vi "流程固件设置对话框.vi"() -> ()   [LabVIEW 2022 SP3, in "斯坦道CODcr.lvlib"]
uses:
  <vilib>/Utility/miscctls.llb/LVPointTypeDef.ctl
panel:
  in  "关键参数查询":bool
  in  "仪器公式":bool
  in  "备用系数":bool
  in  "关闭心跳包":bool
  in  "参数设置":bool
  in  "修改系列号":bool
  in  "关闭":bool
  in  "外设设置":bool
  in  "固件升级":bool
  in  "流程写入":bool
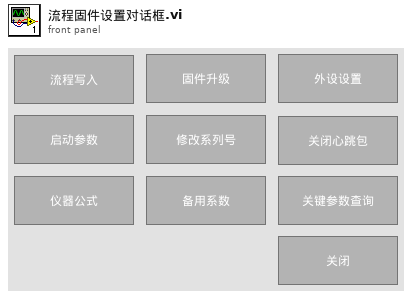
[diagram p1: front panel]
types:
  T1 = enum32{"Invalid", "Standard", "Closed", "Hidden", "Minimized", "Maximized"}
  T2 = typedef "LVPointTypeDef.ctl" = cluster{"Horizontal":i16, "Vertical":i16}
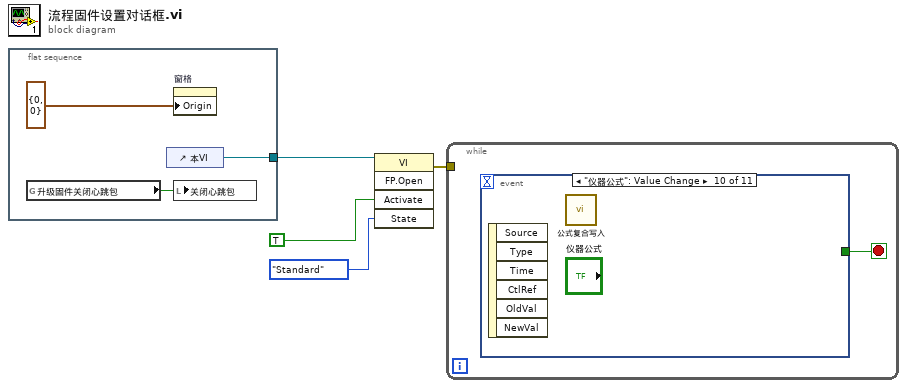
[diagram p0: block diagram]
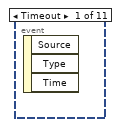
[diagram p2: hidden frame]
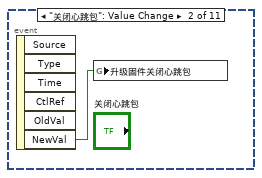
[diagram p3: hidden frame]
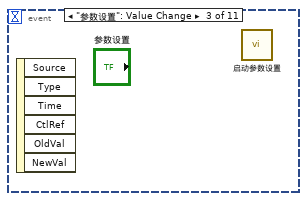
[diagram p4: hidden frame]
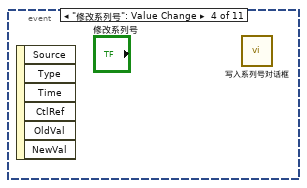
[diagram p5: hidden frame]
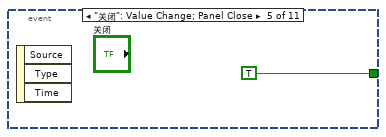
[diagram p6: hidden frame]
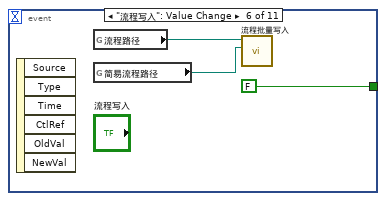
[diagram p7: hidden frame]
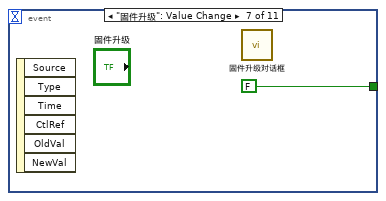
[diagram p8: hidden frame]
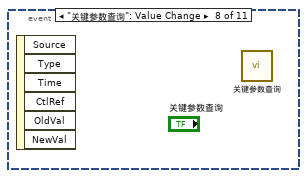
[diagram p9: hidden frame]
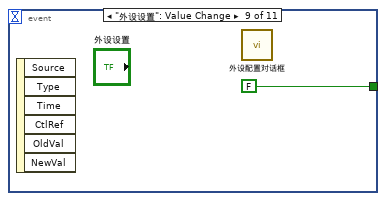
[diagram p10: hidden frame]
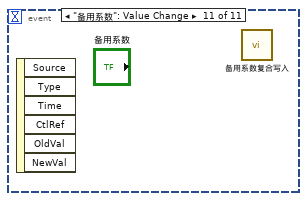
[diagram p11: hidden frame]
diagram:
  n1 = flat-sequence {
    tunnel: [w5] -> w4
    frame #0 {
      n2 = global read "VAR总磷总氮全局变量.vi" "升级固件关闭心跳包"() -> (w6:bool)
      n3 = control-ref of="本VI"() -> (w5:refnum<vi>)
      n4 = property on="窗格" class="Pane"("Origin"=T2 {"Horizontal"=0, "Vertical"=0} ("原点")) -> ()  [unwired: 2 in, 2 out]
      n5 = local write "关闭心跳包"(w6) -> ()
    }
  }
  n6 = invoke class="VI" method="FP.Open"(reference=w4, "Activate"=TRUE ("激活？"), "State"=T1."Standard" ("状态")) -> (error out=w1:errorcluster)  [unwired: 2 in, 4 out]
  n7 = while {
    tunnel: w1 -> [_]
    stop <- w8 stop-if-true
    n8 = event shown="[9] \"仪器公式\": Value Change" {
      selector: _ -> [_ _ _ _ _ _ _ _ _ _ _]
      dyn-events: _ -> [_ _ _ _ _ _ _ _ _ _ _]
      timeout: _ -> [_ _ _ _ _ _ _ _ _ _ _]
      tunnel: [_ _ _ _ TRUE FALSE FALSE _ FALSE _ _] -> w8
      event Timeout {
        n9 = event-data() -> ()  [unwired: 1 in, 3 out]
      }
      event "关闭心跳包": Value Change {
        n10 = event-data() -> ("NewVal"=w9:bool)  [unwired: 1 in, 5 out]
        n11 = global write "VAR总磷总氮全局变量.vi" "升级固件关闭心跳包"(w9) -> ()
      }
      event "参数设置": Value Change {
        n12 = event-data() -> ()  [unwired: 1 in, 6 out]
        n13 = call "启动参数设置.vi"() -> ()  [unwired: 12 in]
      }
      event "修改系列号": Value Change {
        n14 = event-data() -> ()  [unwired: 1 in, 6 out]
        n15 = call "写入系列号对话框.vi"() -> ()  [unwired: 12 in]
      }
      event "关闭": Value Change; Panel Close {
        n16 = event-data() -> ()  [unwired: 1 in, 3 out]
      }
      event "流程写入": Value Change {
        n17 = event-data() -> ()  [unwired: 1 in, 6 out]
        n18 = global read "总磷总氮断电保存全局变量.vi" "流程路径"() -> (w12:path)
        n19 = global read "总磷总氮断电保存全局变量.vi" "简易流程路径"() -> (w11:path)
        n20 = call "流程批量写入.vi"("简易流程路径"=w11, "添加的路径"=w12) -> ()  [unwired: 10 in]
      }
      event "固件升级": Value Change {
        n21 = event-data() -> ()  [unwired: 1 in, 6 out]
        n22 = call "固件升级对话框.vi"() -> ()  [unwired: 12 in]
      }
      event "关键参数查询": Value Change {
        n23 = event-data() -> ()  [unwired: 1 in, 6 out]
        n24 = call "关键参数查询.vi"() -> ()  [unwired: 20 in]
      }
      event "外设设置": Value Change {
        n25 = event-data() -> ()  [unwired: 1 in, 6 out]
        n26 = call "外设配置对话框.vi"() -> ()  [unwired: 12 in]
      }
      event "仪器公式": Value Change {
        n27 = event-data() -> ()  [unwired: 1 in, 6 out]
        n28 = call "公式复合写入.vi"() -> ()  [unwired: 12 in]
      }
      event "备用系数": Value Change {
        n29 = event-data() -> ()  [unwired: 1 in, 6 out]
        n30 = call "备用系数复合写入.vi"() -> ()  [unwired: 12 in]
      }
    }
  }
